vi "Subtract_RexPix_Quad.vi"(7 "Array side":u16(ring) items=["Left", "Bottom", "Right", "Top"], 10 "Num Ref Pix":i32=5, 11 "Quad array":i32[][](array[numeric])=[[1, 2, 3, 4, 5, 100, 200, 300, 600, 600, 600, 600, 600, 900, 600, 600, 600, 600, 600, 600, 600, 600, 600, 600, 600, 600, 600, 600, 600, 600, 600, 600, 600, 600, 600, 600, 600, 600, 600, 600, 600, 600, 600, 600, 600, 600, 600, 600, 600, 600, 600, 600, 600, 600, 600, 600, 600, 600, 600, 600, 600, 600, 600, 600, 600, 600, 600, 600, 600, 600, 600, 600, 600, 600, 600, 600, 600, 600, 600, 600, 600, 600, 600, 600, 600, 600, 600, 600, 600, 600, 600, 600, 600, 600, 600, 600, 600, 600, 600, 600, 600, 600, 600, 600, 600, 600, 600, 600, 600, 600, 600, 600, 600, 600, 600, 600, 600, 600, 600, 600, 600, 600, 600, 600, 600, 600, 600, 600, 600, 600, 600, 600, 600, 600, 600, 600, 600, 600, 600, 600, 600, 600, 600, 600, 600, 600, 600, 600, 600, 600, 600, 600, 600, 600, 600, 600, 600, 600, 600, 600, 600, 600, 600, 600, 600, 600, 600, 600, 600, 600, 600, 600, 600, 600, 600, 600, 600, 600, 600, 600, 600, 600, 600, 600, 600, 600, 600, 600, 600, 600, 600, 600, 600, 600, 600, 600, 600, 600, 600, 600, 600, 600, 600, 600, 600, 600, 600, 600, 600, 600, 600, 600, 600, 600, 600, 600, 600, 600, 600, 600, 600, 600, 600, 600, 600, 600, 600, 600, 600, 600, 600, 600, 600, 600, 600, 600, 600, 600, 600, 600, 600, 600, 600, 600, 600, 600, 600, 600, 600, 600, 600, 600, 600, 600, 600, 600, 600, 600, 600, 600, 600, 600, 600, 600, 600, 600, 600, 600, 600, 600, 600, 600, 600, 600, 600, 600, 600, 600, 600, 600, 600, 600, 600, 600, 600, 600, 600, 600, 600, 600, 600, 600, 600, 600, 600, 600, 600, 600, 600, 600, 600, 600, 600, 600, 600, 600, 600, 600, 600, 600, 600, 600, 600, 600, 600, 600, 600, 600, 600, 600, 600, 600, 600, 600, 600, 600, 600, 600, 600, 600, 600, 600, 600, 600, 600, 600, 600, 600, 600, 600, 600, 600, 600, 600, 600, 600, 600, 600, 600, 600, 600, 600, 600, 600, 600, 600, 600, 600, 600, 600, 600, 600, 600, 600, 600, 600, 600, 600, 600, 600, 600, 600, 600, 600, 600, 600, 600, 600, 600, 600, 600, 600, 600, 600, 600, 600, 600, 600, 600, 600, 600, 600, 600, 600, 600, 600, 600, 600, 600, 600, 600, 600, 600, 600, 600, 600, 600, 600, 600, 600, 600, 600, 600, 600, 600, 600, 600, 600, 600, 600, 600, 600, 600, 600, 600, 600, 600, 600, 600, 600, 600, 600, 600, 600, 600, 600, 600, 600, 600, 600, 600, 600, 600, 600, 600, 600, 600, 600, 600, 600, 600, 600, 600, 600, 600, 600, 600, 600, 600, 600, 600, 600, 600, 600, 600, 600, 600, 600, 600, 600, 600, 600, 600, 600, 600, 600, 600, 600, 600, 600, 600, 600, 600, 600, 600, 600, 600, 600, 600, 600, 600, 600, 600, 600, 600, 600, 600, 600, 600, 600, 600, 600, 600, 600, 600, 600, 600, 600, 600, 600, 600, 600, 600, 600, 600, 600, 600, 600, 600, 600, 600, 600, 600, 600, 600, 600, 600, 600, 600, 600, 600, 600, 600, 600, 600, 600, 600, 600, 600, 600, 600, 600, 600, 600, 600, 600, 600, 600, 600, 600, 600, 600, 600, 600, 600, 600, 600, 600, 600, 600, 600, 600, 600, 600, 600, 600, 600, 600, 600, 600, 600, 600, 600, 600, 600, 600, 600, 600, 600, 600, 600, 600, 600, 600, 600, 600, 600, 600, 600, 600, 600, 600, 600, 600, 600, 600, 600, 600, 600, 600, 600, 600, 600, 600, 600, 600, 600, 600, 600, 600, 600, 600, 600, 600, 600, 600, 600, 600, 600, 600, 600, 600, 600, 600, 600, 600, 600, 600, 600, 600, 600, 600, 600, 600, 600, 600, 600, 600, 600, 600, 600, 600, 600, 600, 600, 600, 600, 600, 600, 600, 600, 600, 600, 600, 600, 600, 600, 600, 600, 600, 600, 600, 600, 600, 600, 600, 600, 600, 600, 600, 600, 600, 600, 600, 600, 600, 600, 600, 600, 600, 600, 600, 600, 600, 600, 600, 600, 600, 600, 600, 600, 600, 600, 600, 600, 600, 600, 600, 600, 600, 600, 600, 600, 600, 600, 600, 600, 600, 600, 600, 600, 600, 600, 600, 600, 600, 600, 600, 600, 600, 600, 600, 600, 600, 600, 600, 600, 600, 600, 600, 600, 600, 600, 600, 600, 600, 600, 600, 600, 600, 600, 600, 600, 600, 600, 600, 600, 600, 600, 600, 600, 600, 600, 600, 600, 600, 600, 600, 600, 600, 600, 600, 600, 600, 600, 600, 600, 600, 600, 600, 600, 600, 600, 600, 600, 600, 600, 600, 600, 600, 600, 600, 600, 600, 600, 600, 600, 600, 600, 600, 600, 600, 600, 600, 600, 600, 600, 600, 600, 600, 600, 600, 600, 600, 600, 600, 600, 600, 600, 600, 600, 600, 600, 600, 600, 600, 600, 600, 600, 600, 600, 600, 600, 600, 600, 600, 600, 600, 600, 600, 600, 600, 600, 600, 600, 600, 600, 600, 600, 600, 600, 600, 600, 600, 600, 600, 600, 600, 600, 600, 600, 600, 600, 600, 600, 600, 600, 600, 600, 600, 600, 600, 600, 600, 600, 600, 600, 600, 600, 600, 600, 600, 600, 600, 600, 600, 600, 600, 600, 600, 600, 600, 600, 600, 600, 600, 600, 600, 600, 600, 600, 600, 600, 600, 600, 600, 600, 600, 600, 600, 600, 600, 600, 600, 600, 600, 600, 600, 600, 600, 600, 600, 600, 600, 600, 600, 600, 600, 600, 600, 600, 600, 600, 600, 600, 600, 600, 600, 600, 600, 600, 600, 600, 600, 600, 600, 600, 600, 600, 600, 600, 600, 600, 600, 600, 600, 600, 600, 600, 600, 600, 600, 600, 600, 600, 600, 600, 600, 600, 600, 600, 600, 600, 600, 600, 600, 600, 600, 600, 600, 600, 600, 600, 600, 600, 600, 600, 600, 600, 600, 600, 600, 600, 600, 600, 600, 600, 600, 600, 600, 600, 600, 600, 600, 600, 600, 600, 600, 600, 600, 600, 600, 600, 600, 600, 600, 600, 600, 600, 600, 600, 600, 600, 600, 600, 600, 800, 900, 1000, -1, -2, -3, -4, -5], [1, 2, 3, 0, 0, 400, 500, 600, 600, 600, 600, 600, 600, 600, 600, 600, 600, 600, 600, 600, 600, 600, 600, 600, 600, 600, 600, 600, 600, 600, 600, 600, 600, 600, 600, 600, 600, 600, 600, 600, 600, 600, 600, 600, 600, 600, 600, 600, 600, 600, 600, 600, 600, 600, 600, 600, 600, 600, 600, 600, 600, 600, 600, 600, 600, 600, 600, 600, 600, 600, 600, 600, 600, 600, 600, 600, 600, 600, 600, 600, 600, 600, 600, 600, 600, 600, 600, 600, 600, 600, 600, 600, 600, 600, 600, 600, 600, 600, 600, 600, 600, 600, 600, 600, 600, 600, 600, 600, 600, 600, 600, 600, 600, 600, 600, 600, 600, 600, 600, 600, 600, 600, 600, 600, 600, 600, 600, 600, 600, 600, 600, 600, 600, 600, 600, 600, 600, 600, 600, 600, 600, 600, 600, 600, 600, 600, 600, 600, 600, 600, 600, 600, 600, 600, 600, 600, 600, 600, 600, 600, 600, 600, 600, 600, 600, 600, 600, 600, 600, 600, 600, 600, 600, 600, 600, 600, 600, 600, 600, 600, 600, 600, 600, 600, 600, 600, 600, 600, 600, 600, 600, 600, 600, 600, 600, 600, 600, 600, 600, 600, 600, 600, 600, 600, 600, 600, 600, 600, 600, 600, 600, 600, 600, 600, 600, 600, 600, 600, 600, 600, 600, 600, 600, 600, 600, 600, 600, 600, 600, 600, 600, 600, 600, 600, 600, 600, 600, 600, 600, 600, 600, 600, 600, 600, 600, 600, 600, 600, 600, 600, 600, 600, 600, 600, 600, 600, 600, 600, 600, 600, 600, 600, 600, 600, 600, 600, 600, 600, 600, 600, 600, 600, 600, 600, 600, 600, 600, 600, 600, 600, 600, 600, 600, 600, 600, 600, 600, 600, 600, 600, 600, 600, 600, 600, 600, 600, 600, 600, 600, 600, 600, 600, 600, 600, 600, 600, 600, 600, 600, 600, 600, 600, 600, 600, 600, 600, 600, 600, 600, 600, 600, 600, 600, 600, 600, 600, 600, 600, 600, 600, 600, 600, 600, 600, 600, 600, 600, 600, 600, 600, 600, 600, 600, 600, 600, 600, 600, 600, 600, 600, 600, 600, 600, 600, 600, 600, 600, 600, 600, 600, 600, 600, 600, 600, 600, 600, 600, 600, 600, 600, 600, 600, 600, 600, 600, 600, 600, 600, 600, 600, 600, 600, 600, 600, 600, 600, 600, 600, 600, 600, 600, 600, 600, 600, 600, 600, 600, 600, 600, 600, 600, 600, 600, 600, 600, 600, 600, 600, 600, 600, 600, 600, 600, 600, 600, 600, 600, 600, 600, 600, 600, 600, 600, 600, 600, 600, 600, 600, 600, 600, 600, 600, 600, 600, 600, 600, 600, 600, 600, 600, 600, 600, 600, 600, 600, 600, 600, 600, 600, 600, 600, 600, 600, 600, 600, 600, 600, 600, 600, 600, 600, 600, 600, 600, 600, 600, 600, 600, 600, 600, 600, 600, 600, 600, 600, 600, 600, 600, 600, 600, 600, 600, 600, 600, 600, 600, 600, 600, 600, 600, 600, 600, 600, 600, 600, 600, 600, 600, 600, 600, 600, 600, 600, 600, 600, 600, 600, 600, 600, 600, 600, 600, 600, 600, 600, 600, 600, 600, 600, 600, 600, 600, 600, 600, 600, 600, 600, 600, 600, 600, 600, 600, 600, 600, 600, 600, 600, 600, 600, 600, 600, 600, 600, 600, 600, 600, 600, 600, 600, 600, 600, 600, 600, 600, 600, 600, 600, 600, 600, 600, 600, 600, 600, 600, 600, 600, 600, 600, 600, 600, 600, 600, 600, 600, 600, 600, 600, 600, 600, 600, 600, 600, 600, 600, 600, 600, 600, 600, 600, 600, 600, 600, 600, 600, 600, 600, 600, 600, 600, 600, 600, 600, 600, 600, 600, 600, 600, 600, 600, 600, 600, 600, 600, 600, 600, 600, 600, 600, 600, 600, 600, 600, 600, 600, 600, 600, 600, 600, 600, 600, 600, 600, 600, 600, 600, 600, 600, 600, 600, 600, 600, 600, 600, 600, 600, 600, 600, 600, 600, 600, 600, 600, 600, 600, 600, 600, 600, 600, 600, 600, 600, 600, 600, 600, 600, 600, 600, 600, 600, 600, 600, 600, 600, 600, 600, 600, 600, 600, 600, 600, 600, 600, 600, 600, 600, 600, 600, 600, 600, 600, 600, 600, 600, 600, 600, 600, 600, 600, 600, 600, 600, 600, 600, 600, 600, 600, 600, 600, 600, 600, 600, 600, 600, 600, 600, 600, 600, 600, 600, 600, 600, 600, 600, 600, 600, 600, 600, 600, 600, 600, 600, 600, 600, 600, 600, 600, 600, 600, 600, 600, 600, 600, 600, 600, 600, 600, 600, 600, 600, 600, 600, 600, 600, 600, 600, 600, 600, 600, 600, 600, 600, 600, 600, 600, 600, 600, 600, 600, 600, 600, 600, 600, 600, 600, 600, 600, 600, 600, 600, 600, 600, 600, 600, 600, 600, 600, 600, 600, 600, 600, 600, 600, 600, 600, 600, 600, 600, 600, 600, 600, 600, 600, 600, 600, 600, 600, 600, 600, 600, 600, 600, 600, 600, 600, 600, 600, 600, 600, 600, 600, 600, 600, 600, 600, 600, 600, 600, 600, 600, 600, 600, 600, 600, 600, 600, 600, 600, 600, 600, 600, 600, 600, 600, 600, 600, 600, 600, 600, 600, 600, 600, 600, 600, 600, 600, 600, 600, 600, 600, 600, 600, 600, 600, 600, 600, 600, 600, 600, 600, 600, 600, 600, 600, 600, 600, 600, 600, 600, 600, 600, 600, 600, 600, 600, 600, 600, 600, 600, 600, 600, 600, 600, 600, 600, 600, 600, 600, 600, 600, 600, 600, 600, 600, 600, 600, 600, 600, 600, 600, 600, 600, 600, 600, 600, 600, 600, 600, 600, 600, 600, 600, 600, 600, 600, 600, 600, 600, 600, 600, 600, 600, 600, 600, 600, 600, 600, 600, 600, 600, 600, 600, 600, 600, 600, 600, 600, 600, 600, 600, 600, 600, 600, 600, 600, 600, 600, 600, 600, 600, 600, 600, 600, 600, 600, 600, 600, 600, 600, 600, 600, 600, 600, 600, 600, 600, 600, 600, 600, 600, 600, 600, 600, 600, 600, 600, 600, 600, 600, 600, 600, 600, 600, 600, 600, 600, 600, 600, 600, 600, 600, 600, 600, 600, 600, 600, 600, 600, 600, 600, 600, 600, 600, 600, 600, 600, 600, 600, 600, 600, -10, -20, -30, -40, -50]]) -> (0 "RMS 2":dbl, 1 "mean 2":dbl, 2 "Avg ref pixels":dbl[](array[numeric]), 3 "Quad array subtracted ref pixs":i32[][](array[numeric]))   [LabVIEW 2017]
panel:
  out "IMAGE 3":i32[][](graph)
  out "Sub pxis sel array":i32[][](array[numeric])
  out "IMAGE 2":i32[][](graph)
  out "RMS":dbl
  out "mean":dbl
  out "IMAGE":dbl[][](graph)
  out "Ref pix array size":i32
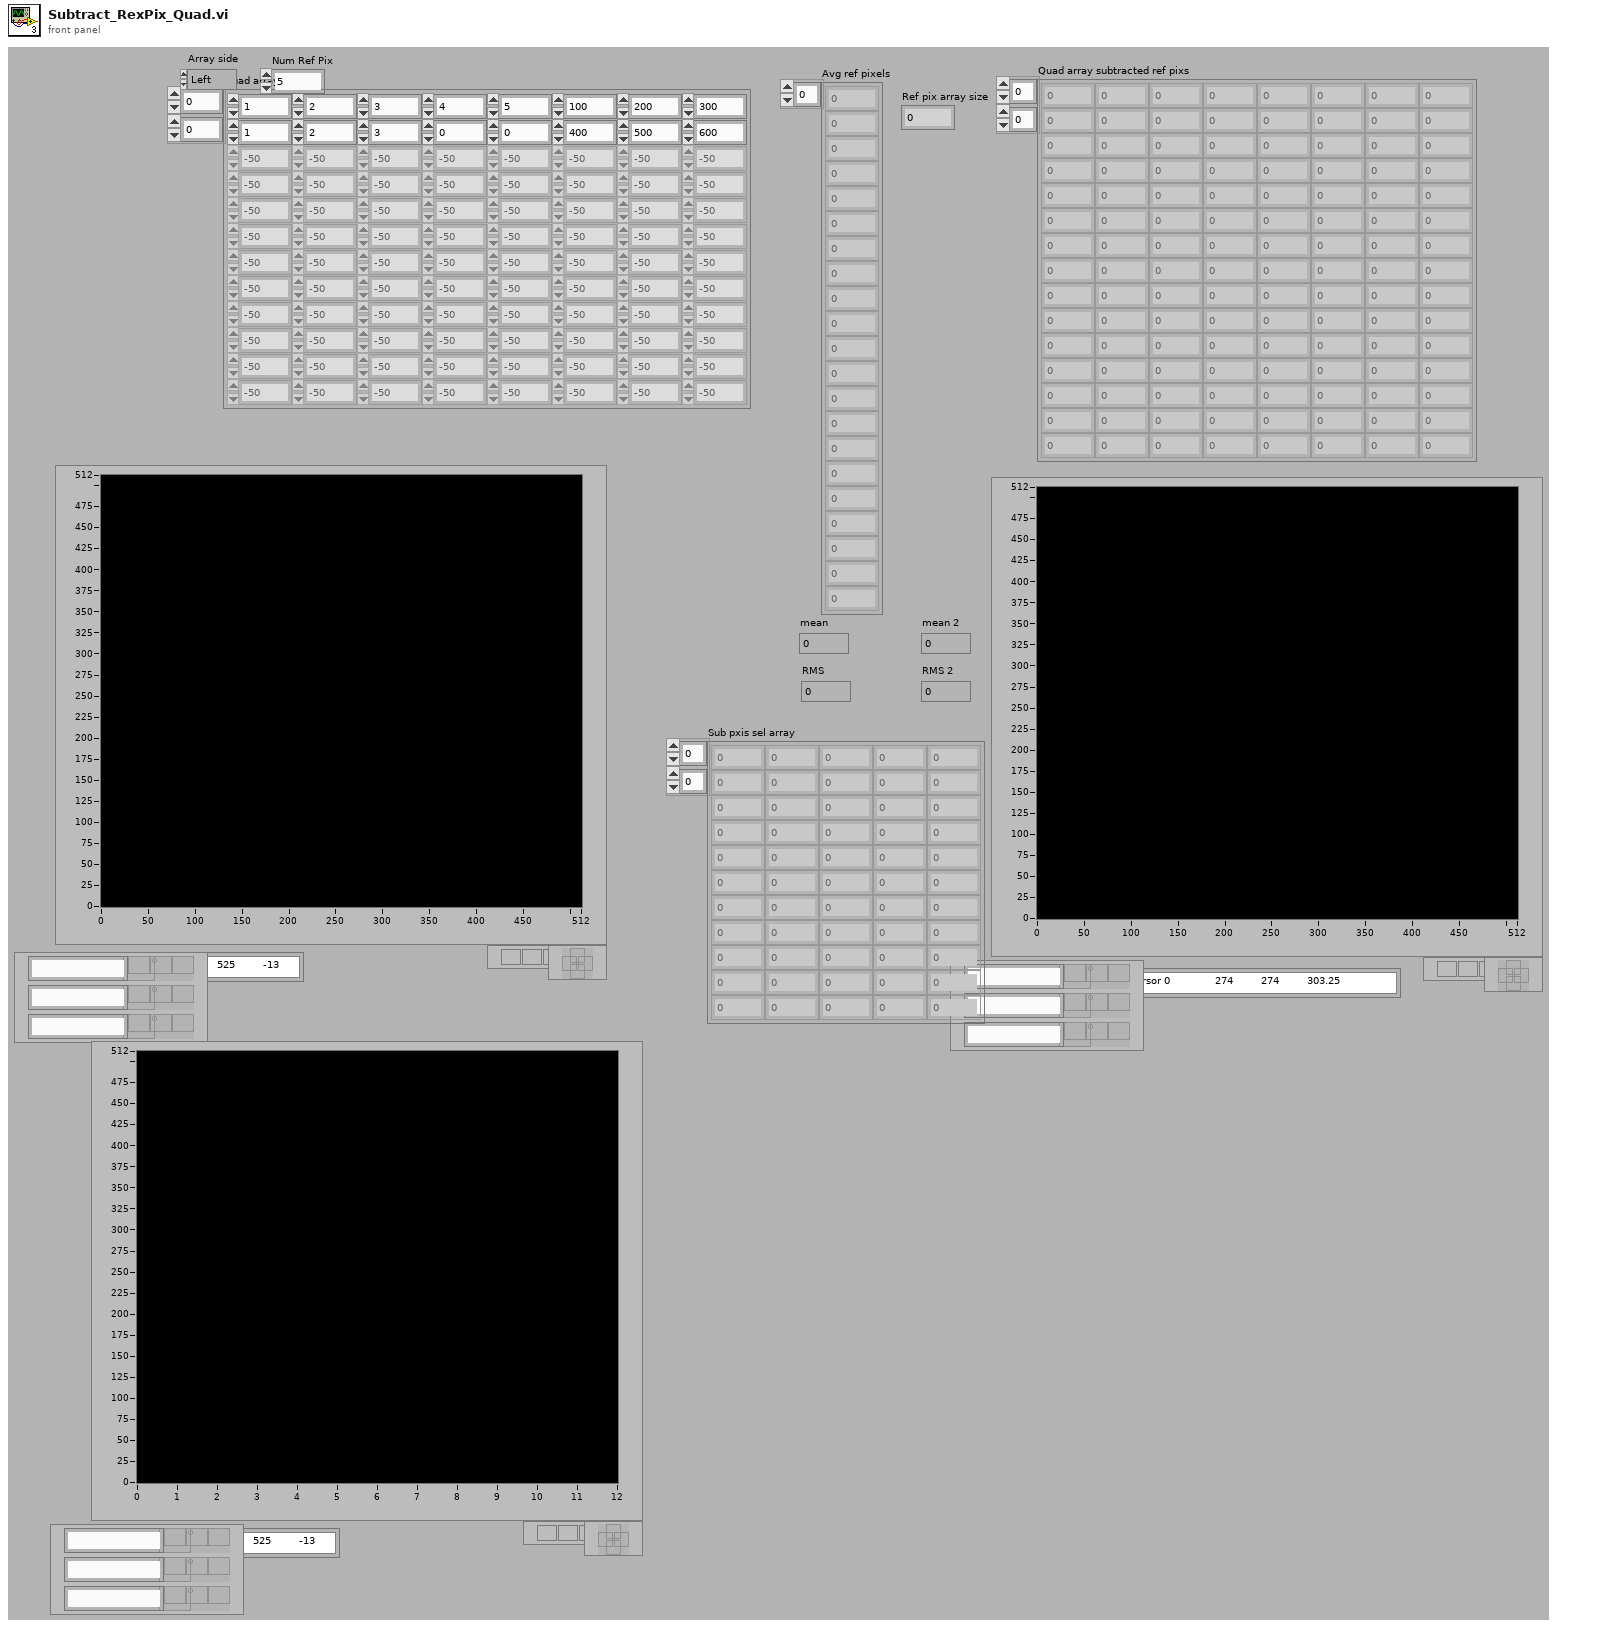
[diagram p1: front panel]
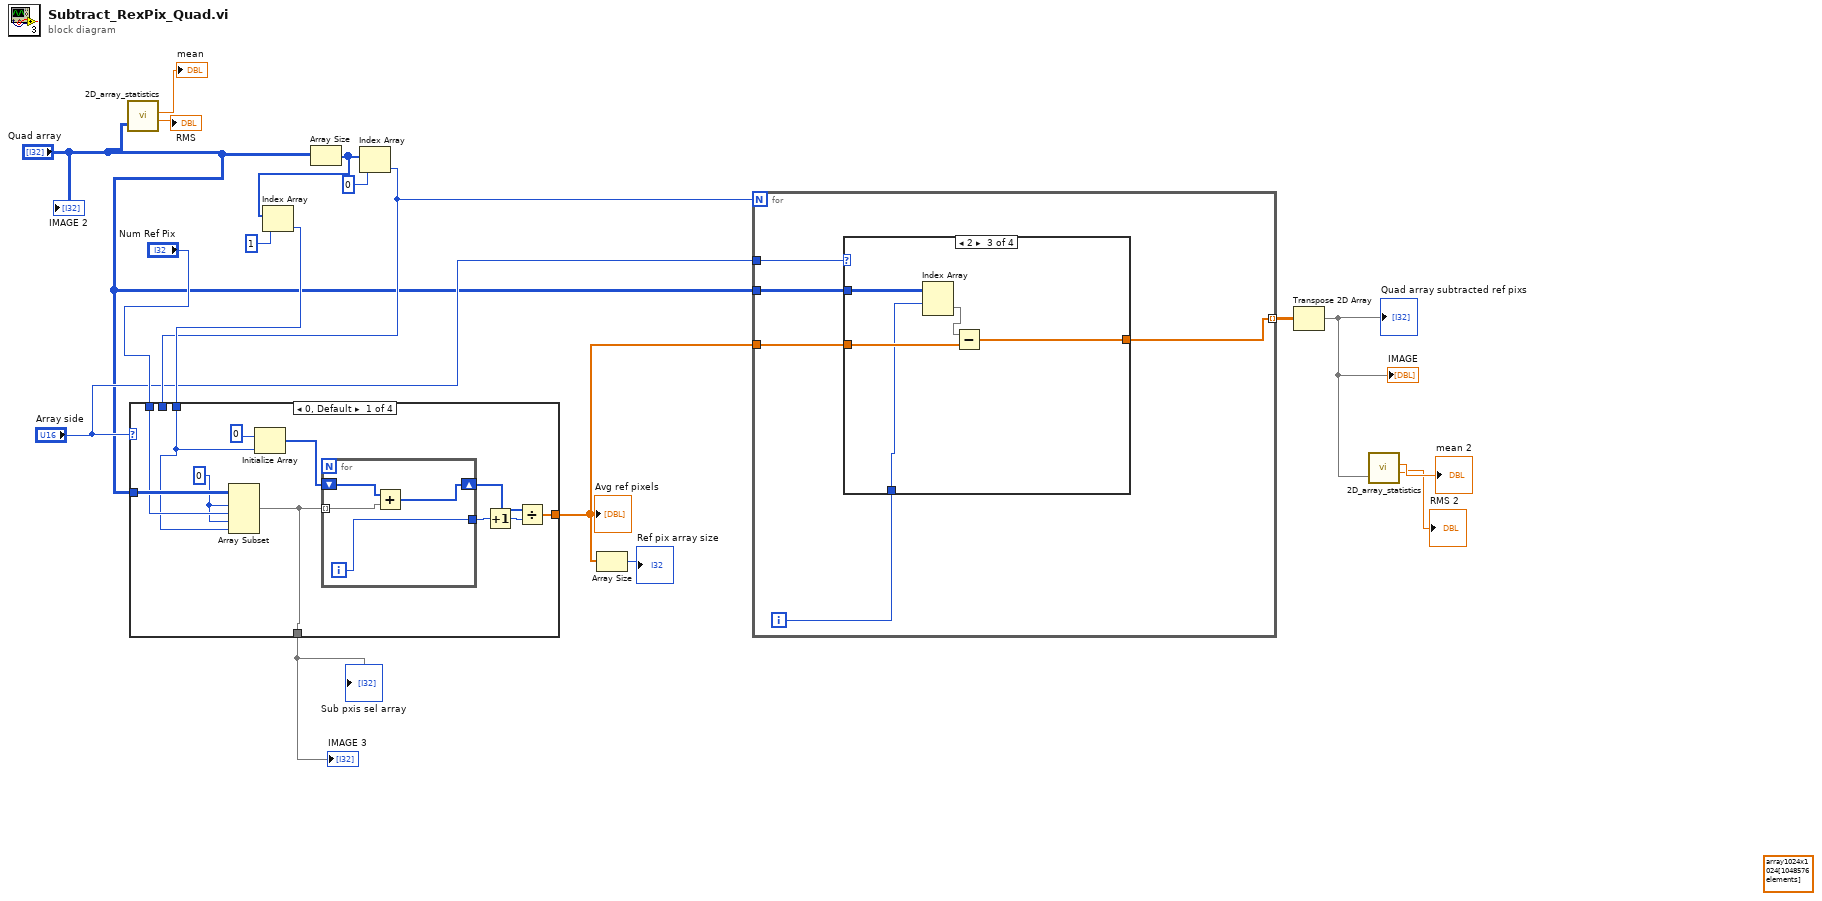
[diagram p0: block diagram]
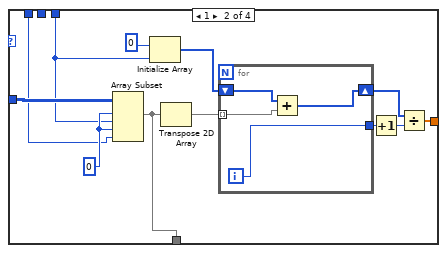
[diagram p2: hidden frame]
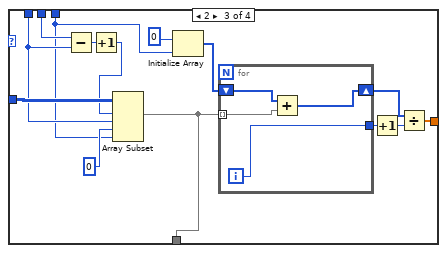
[diagram p3: hidden frame]
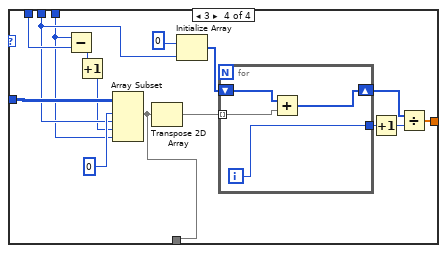
[diagram p4: hidden frame]
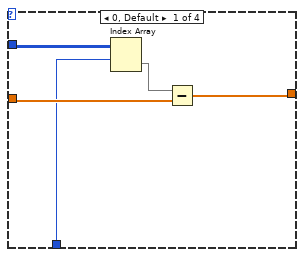
[diagram p5: hidden frame]
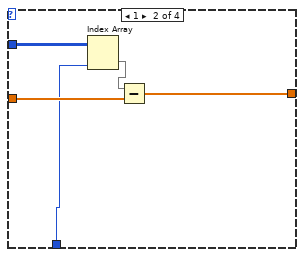
[diagram p6: hidden frame]
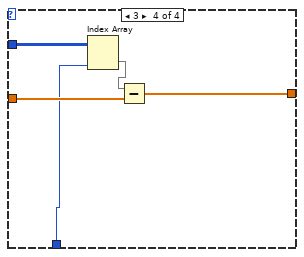
[diagram p7: hidden frame]
diagram:
  (unwired) dbl[][] array1024x1024[1048576 elements] ("IMAGE")
  n1 = call <userlib>:"2D_array_statistics.vi"("Array"="Quad array") -> ("mean 2"=→"mean":dbl, "RMS 2"=→"RMS":dbl)  [unwired: 2 in, 2 out]
  n2 = Array Size(array="Quad array") -> (size(s)=w15:i32[])
  n3 = Index Array(array=w15, index=1) -> (element=w14:i32)
  n4 = Index Array(array=w15, index=0) -> (element=w13:i32)
  n5 = case shown="0, Default" "Array side" {
    tunnel: "Quad array" -> [w28 w44 w62 w81]
    tunnel: "Num Ref Pix" -> [w27 w42 w57 w74]
    tunnel: w14 -> [w20 w36 w54 w71]
    tunnel: w13 -> [_ _ w56 w72]
    tunnel: [w23 w39 w58 w78] -> w10
    tunnel: [w18 w33 w51 w69] -> w1
    frame 0, Default {
      w26 = 0 ("index")
      n6 = Array Subset(array=w28, index (row)=w26, length (row)=w27, index (col)=w26, length (col)=w20) -> (w18:i32[][])
      n7 = Initialize Array(0, w20) -> (w21:i32[])
      n8 = for {
        tunnel: w18 -> [w32] mode=indexing
        shift-right: [w30] -> w25
        shift-left: w21 -> [w31]
        tunnel: [w29] -> w24
        i -> [w29]
        n9 = Add(x=w31, y=w32) -> (x+y=w30:i32[])
      }
      n10 = Increment(x=w24) -> (x+1=w19:i32)
      n11 = Divide(x=w25, y=w19) -> (x/y=w23:dbl[])
    }
    frame 1 {
      w43 = 0 ("index")
      n12 = Array Subset(array=w44, index (row)=w43, length (row)=w36, index (col)=w43, length (col)=w42) -> (w33:i32[][])
      n13 = Initialize Array(0, w36) -> (w37:i32[])
      n14 = Transpose 2D Array(2D array=w33) -> (transposed array=w34:i32[][])
      n15 = for {
        tunnel: w34 -> [w48] mode=indexing
        shift-right: [w46] -> w41
        shift-left: w37 -> [w47]
        tunnel: [w45] -> w40
        i -> [w45]
        n16 = Add(x=w47, y=w48) -> (x+y=w46:i32[])
      }
      n17 = Increment(x=w40) -> (x+1=w35:i32)
      n18 = Divide(x=w41, y=w35) -> (x/y=w39:dbl[])
    }
    frame 2 {
      n19 = Subtract(x=w56, y=w57) -> (x-y=w50:i32)
      n20 = Increment(x=w50) -> (x+1=w49:i32)
      n21 = Array Subset(array=w62, index (row)=w49, length (row)=w57, index (col)=0 ("index"), length (col)=w54) -> (w51:i32[][])
      n22 = Initialize Array(0, w54) -> (w53:i32[])
      n23 = for {
        tunnel: w51 -> [w66] mode=indexing
        shift-right: [w64] -> w60
        shift-left: w53 -> [w65]
        tunnel: [w63] -> w59
        i -> [w63]
        n24 = Add(x=w65, y=w66) -> (x+y=w64:i32[])
      }
      n25 = Increment(x=w59) -> (x+1=w52:i32)
      n26 = Divide(x=w60, y=w52) -> (x/y=w58:dbl[])
    }
    frame 3 {
      n27 = Subtract(x=w71, y=w74) -> (x-y=w70:i32)
      n28 = Increment(x=w70) -> (x+1=w67:i32)
      n29 = Array Subset(array=w81, index (row)=0 ("index"), length (row)=w72, index (col)=w67, length (col)=w71) -> (w69:i32[][])
      n30 = Transpose 2D Array(2D array=w69) -> (transposed array=w68:i32[][])
      n31 = Initialize Array(0, w72) -> (w75:i32[])
      n32 = for {
        tunnel: w68 -> [w85] mode=indexing
        shift-right: [w83] -> w80
        shift-left: w75 -> [w84]
        tunnel: [w82] -> w79
        i -> [w82]
        n33 = Add(x=w84, y=w85) -> (x+y=w83:i32[])
      }
      n34 = Increment(x=w79) -> (x+1=w73:i32)
      n35 = Divide(x=w80, y=w73) -> (x/y=w78:dbl[])
    }
  }
  "Avg ref pixels" <- w10
  "Sub pxis sel array" <- w1
  "IMAGE 3" <- w1
  n36 = Array Size(array=w10) -> (size(s)=→"Ref pix array size":i32)
  n37 = for {
    N: w13 -> [_]
    tunnel: [w89] -> w6 mode=indexing
    tunnel: "Quad array" -> [w88]
    tunnel: w10 -> [w90]
    tunnel: "Array side" -> [w87]
    i -> [w86]
    n38 = case shown="2" w87 {
      tunnel: w90 -> [w94 w100 w105 w110]
      tunnel: [w92 w99 w104 w109] -> w89
      tunnel: w88 -> [w95 w98 w103 w108]
      tunnel: w86 -> [w91 w97 w101 w107]
      frame 0, Default {
        n39 = Index Array(array=w95, index (row)=w91) -> (element=w93:i32[])  [unwired: 1 in]
        n40 = Subtract(x=w93, y=w94) -> (x-y=w92:dbl[])
      }
      frame 1 {
        n41 = Index Array(array=w98, index (col)=w97) -> (element=w96:i32[])  [unwired: 1 in]
        n42 = Subtract(x=w96, y=w100) -> (x-y=w99:dbl[])
      }
      frame 2 {
        n43 = Index Array(array=w103, index (row)=w101) -> (element=w102:i32[])  [unwired: 1 in]
        n44 = Subtract(x=w102, y=w105) -> (x-y=w104:dbl[])
      }
      frame 3 {
        n45 = Index Array(array=w108, index (col)=w107) -> (element=w106:i32[])  [unwired: 1 in]
        n46 = Subtract(x=w106, y=w110) -> (x-y=w109:dbl[])
      }
    }
  }
  n47 = Transpose 2D Array(2D array=w6) -> (transposed array=w2:dbl[][])
  "Quad array subtracted ref pixs" <- w2
  "IMAGE" <- w2
  n48 = call <userlib>:"2D_array_statistics.vi"("Array"=w2) -> ("mean 2"=→"mean 2":dbl, "RMS 2"=→"RMS 2":dbl)  [unwired: 2 in, 2 out]
  "IMAGE 2" <- "Quad array"
